vi "string concentenate and ramp funciton.vi"() -> ()   [LabVIEW 2024]
uses:
  <vilib>/Analysis/1siggen.llb/Ramp Pattern by Delta.vi
  <vilib>/Analysis/NI_AALBase.lvlib
panel:
  out "Ramp Pattern":dbl[](array[numeric])
  out "concatenated string":string
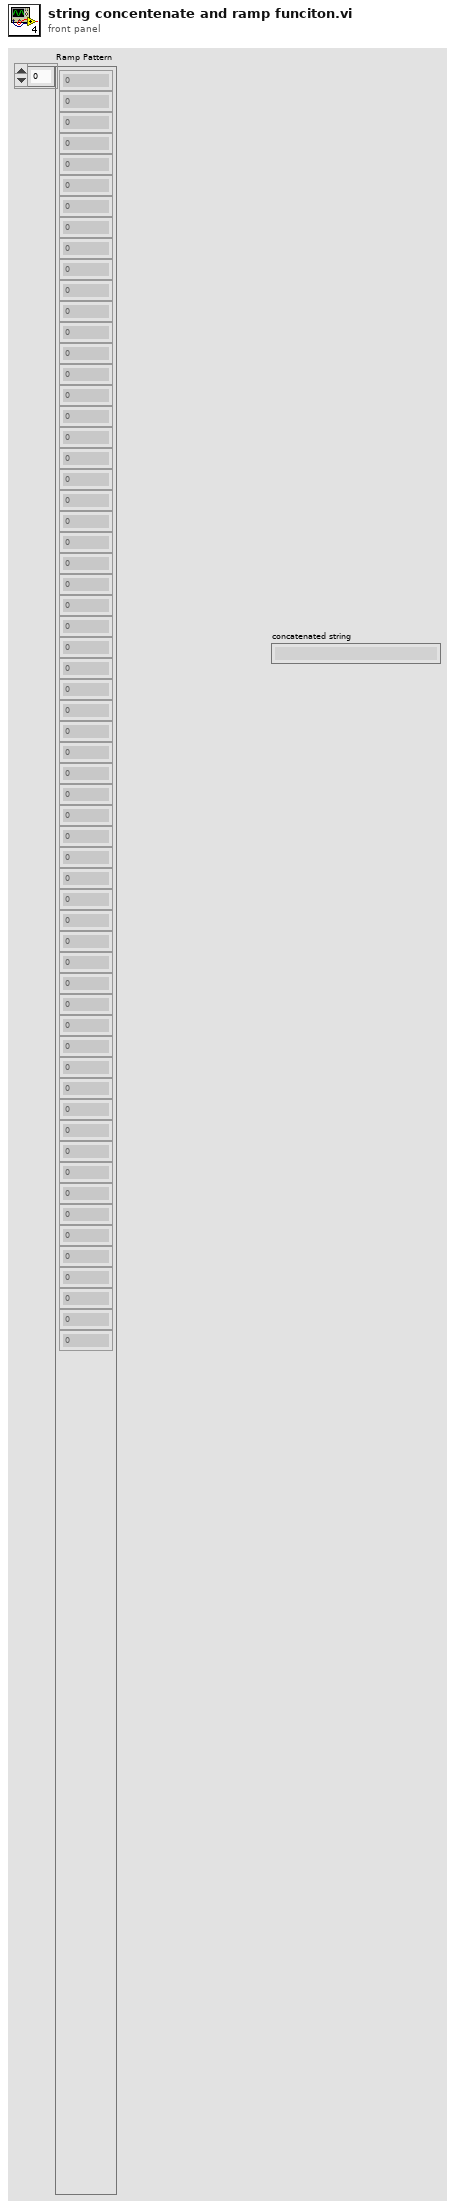
[diagram p1: front panel]
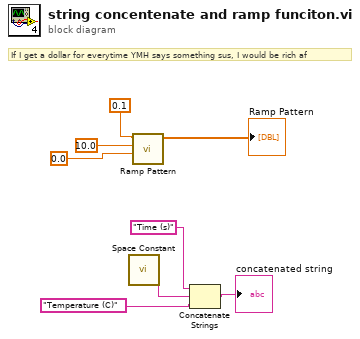
[diagram p0: block diagram]
diagram:
  # "If I get a dollar for everytime YMH says something sus, I would be rich af"
  n1 = call <vilib>:"Space Constant.vi"() -> ("String"=w8:string)
  n2 = call-poly <vilib>:"Ramp Pattern.vi"("start"=0.0, "end"=10.0, "delta"=0.1) -> ("Ramp Pattern"=→"Ramp Pattern":dbl[])  [unwired: 6 in, 2 out]
  n3 = Concatenate Strings("Time (s)" ("string"), w8, "Temperature (C)" ("string")) -> (→"concatenated string":string)
